vi "main.vi"() -> ()   [LabVIEW 2023]
uses:
  Enum.ctl
  typeDef/enum mesure.ctl
  Desktop/Open_device_2018.llb/Select_Instr.ctl
panel:
  in  "VISA resource name":refnum<visa-resource-name>
  out "?":T1
  out "Horizontal Progress Bar":u8(slide) scale=0.0..100.0
  in  "Exit program":bool
  in  "Start measure":bool
  in  "Pause measure":bool
  in  "Save As Button":bool
  in  "Sample distribution for graph":enum32{"Logarytmic", "Linear"}(radio)
  out "XY Graph":cluster{"X":dbl, "Y":dbl}[](graph)
  in  "Sample distribution":enum32{"Logarytmic", "Linear"}(radio)
  in  "Density distribution":dbl
  in  "Amplitude":dbl
  in  "Stop frequency":dbl
  in  "Start frequency":dbl
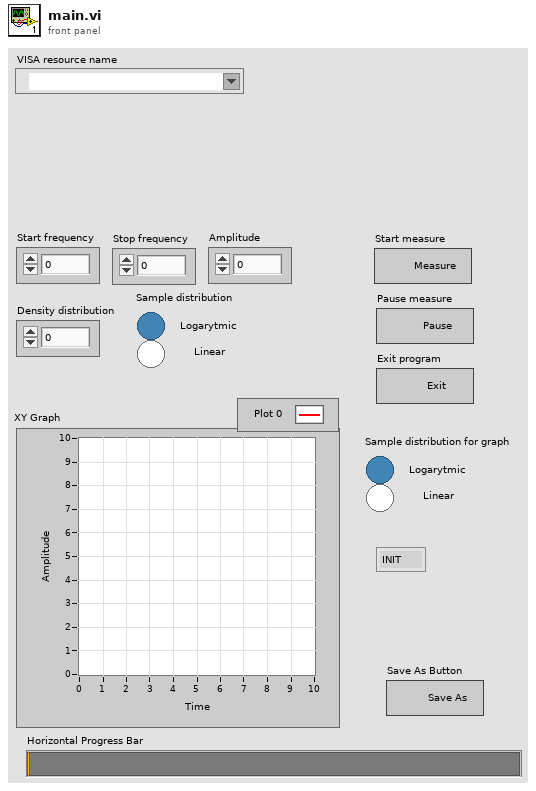
[diagram p1: front panel]
types:
  T1 = typedef "Enum.ctl" = enum16{"INIT", "IDLE", "SAVE", "CONN_TO_DEV", "MEASURE", "END", "CONN_TO_COM"}
  T2 = cluster{"COM_OK":bool, "MEASURE":bool, "komutator":refnum<visa-resource-name>, "generator":refnum<visa-resource-name>, "miernik":refnum<visa-resource-name>}
  T3 = typedef "enum mesure.ctl" = enum16{"Set_gen", "Obj_1", "Obj_2", "Obj_3", "Obj_4", "Obj_5"}
  T4 = typedef "Select_Instr.ctl" = string
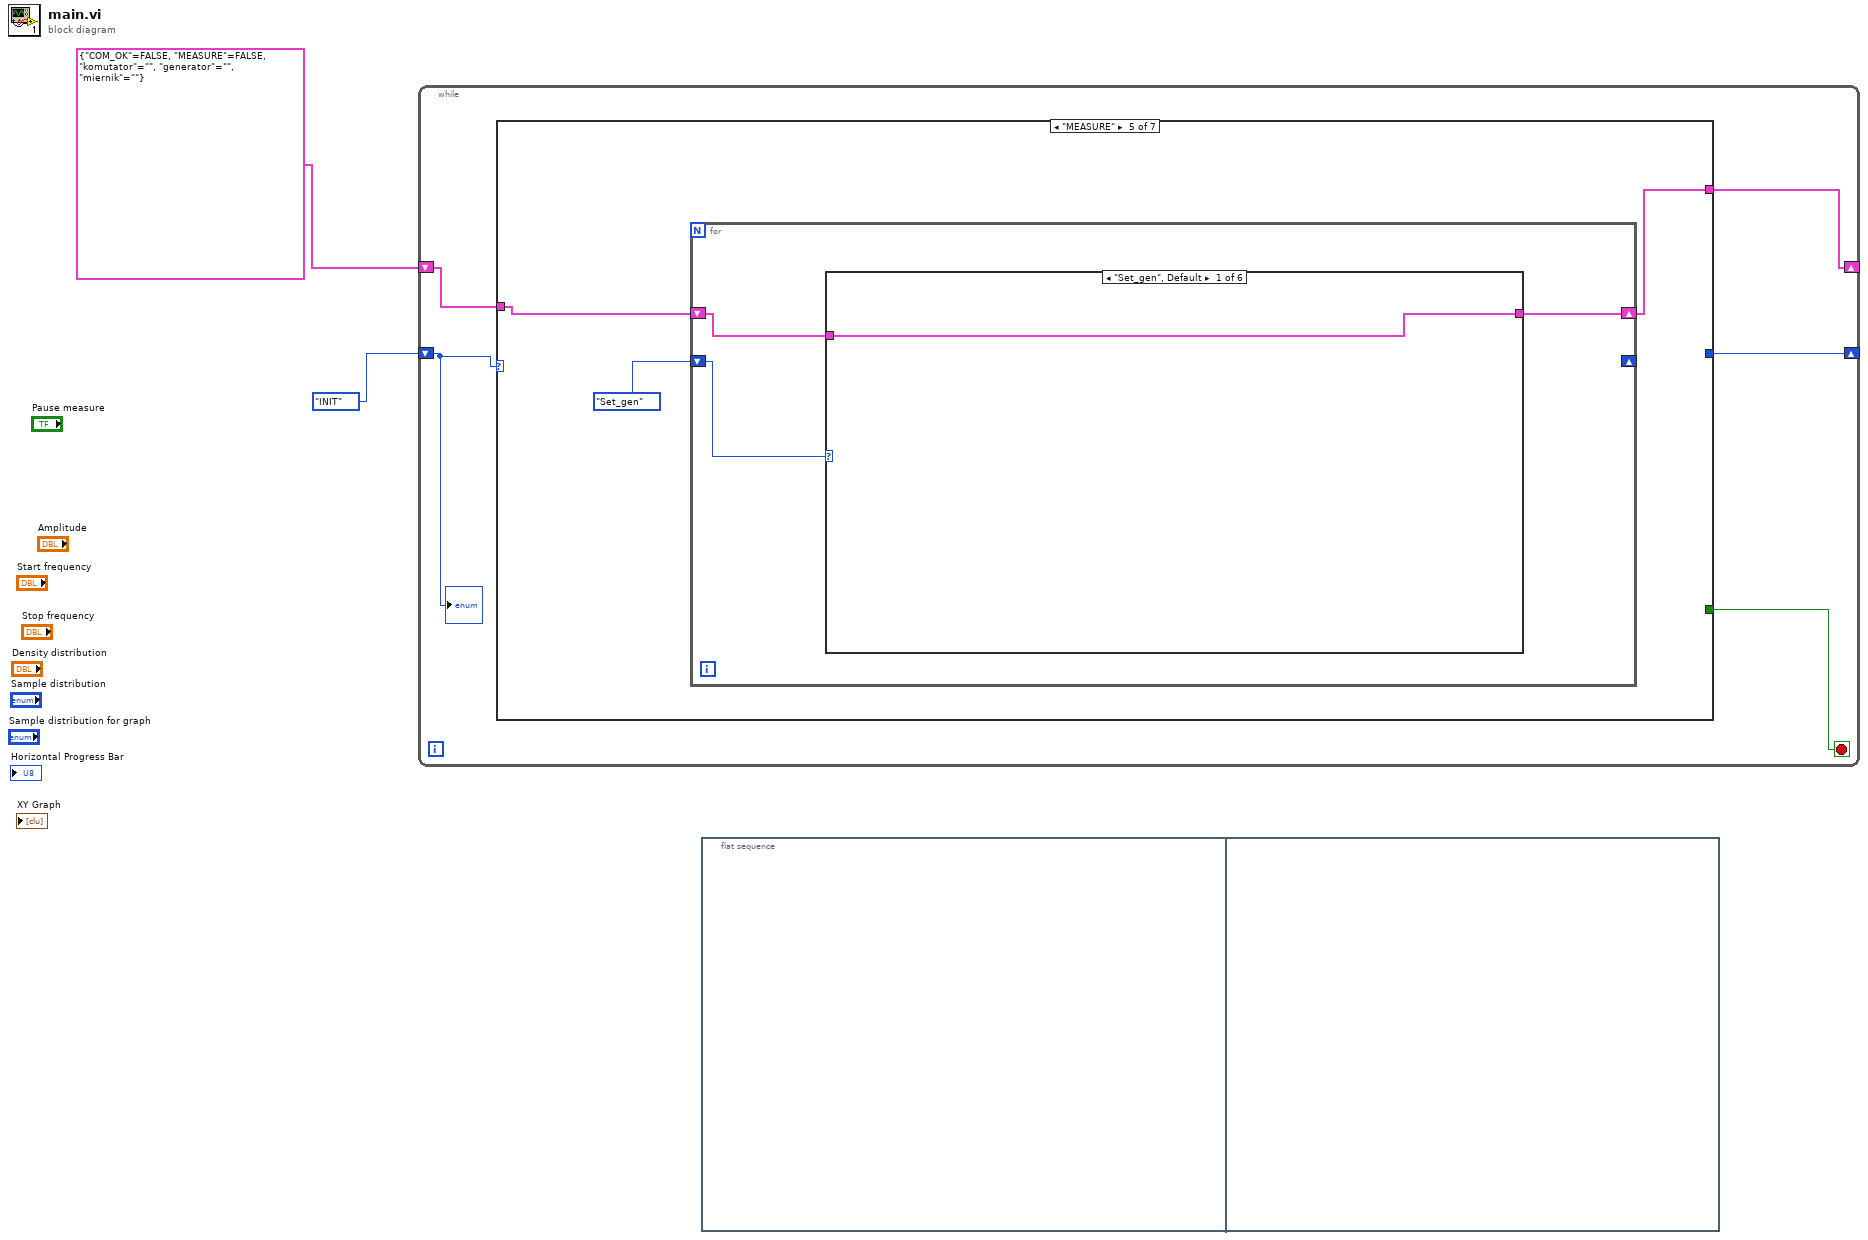
[diagram p0: block diagram]
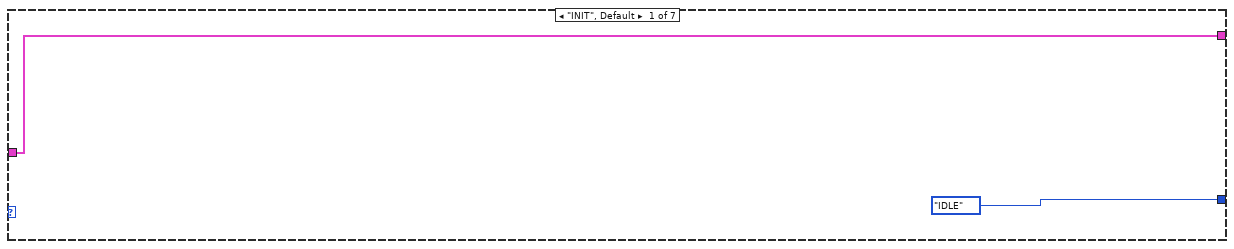
[diagram p2: hidden frame]
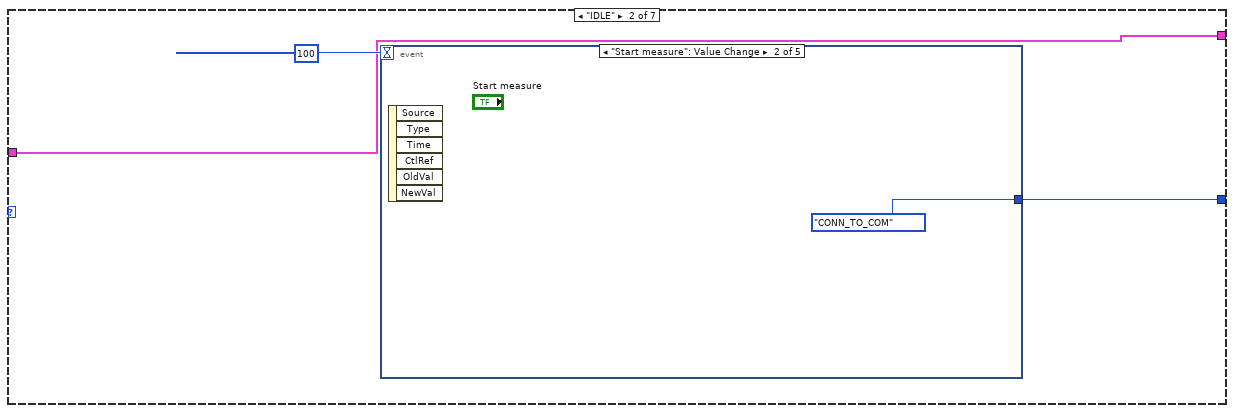
[diagram p3: hidden frame]
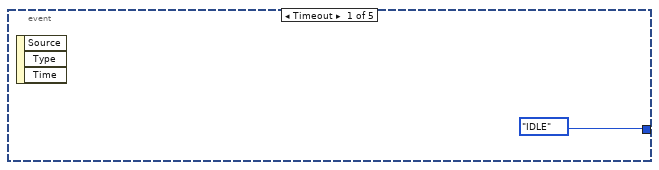
[diagram p4: hidden frame]
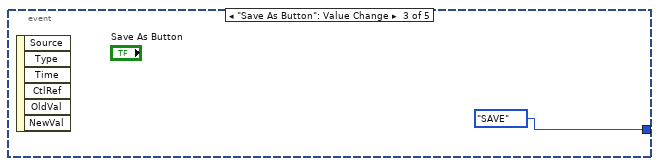
[diagram p5: hidden frame]
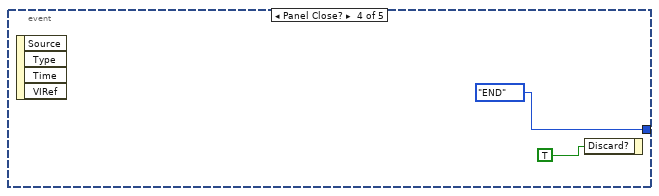
[diagram p6: hidden frame]
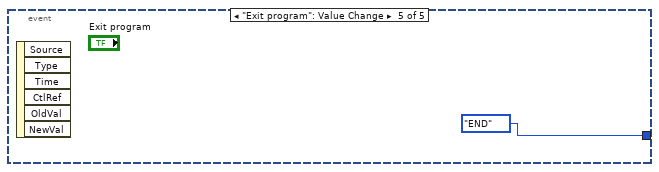
[diagram p7: hidden frame]
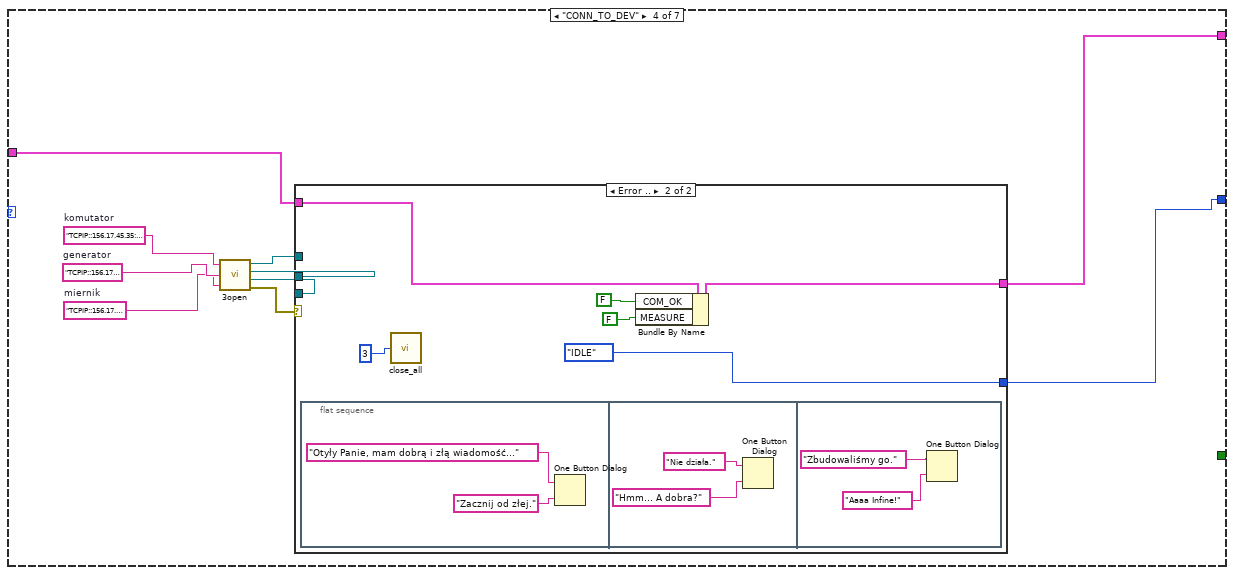
[diagram p9: hidden frame]
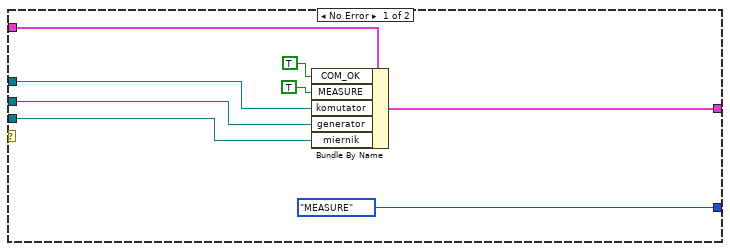
[diagram p10: hidden frame]
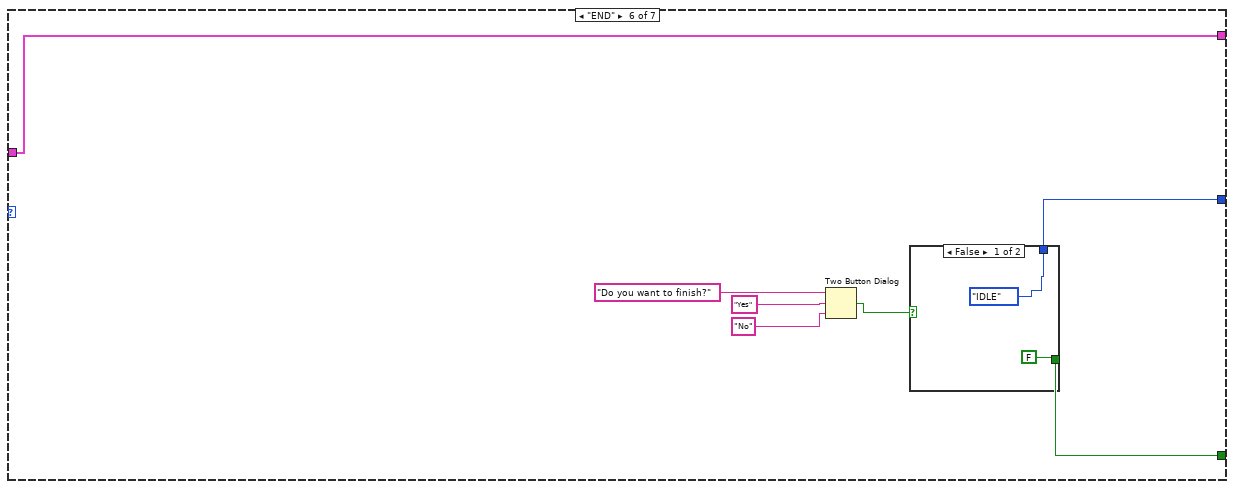
[diagram p16: hidden frame]
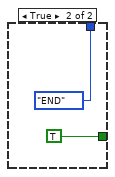
[diagram p17: hidden frame]
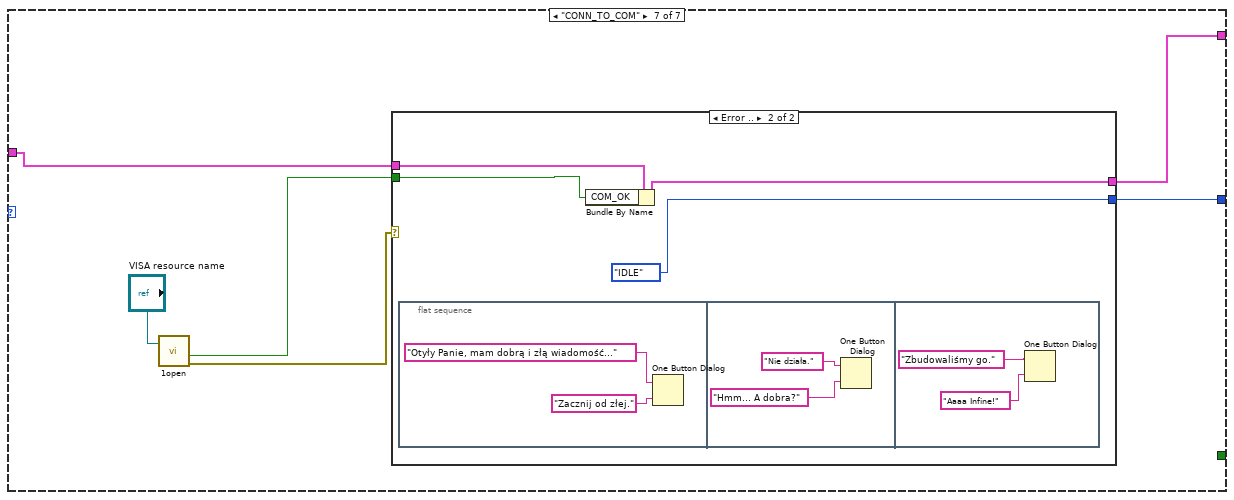
[diagram p18: hidden frame]
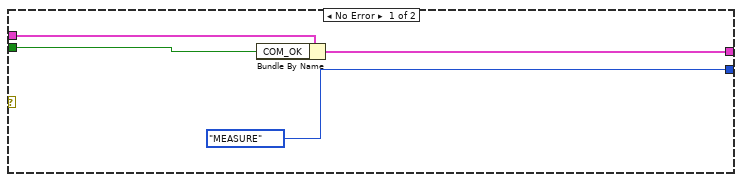
[diagram p19: hidden frame]
diagram:
  n1 = while {
    shift-right: [w5] -> _
    shift-left: Enum."INIT" -> [w7]
    shift-right: [w3] -> _
    shift-left: T2 {"COM_OK"=FALSE, "MEASURE"=FALSE, "komutator"="", "generator"="", "miernik"=""} -> [w4]
    stop <- w6 stop-if-true
    n2 = case shown="\"MEASURE\"" w7 {
      tunnel: [_ _ _ _ _ w59 _] -> w6
      tunnel: [Enum."IDLE" w12 _ w20 _ w58 w68] -> w5
      tunnel: w4 -> [w8 w10 w19 w25 w51 w57 w71]
      tunnel: [w8 w10 w19 w24 w50 w57 w69] -> w3
      frame "INIT", Default {
      }
      frame "IDLE" {
        n3 = event shown="[1] \"Start measure\": Value Change" {
          selector: _ -> [_ _ _ _ _]
          dyn-events: _ -> [_ _ _ _ _]
          timeout: 100 -> [_ _ _ _ _]
          tunnel: [Enum."IDLE" Enum."CONN_TO_COM" Enum."SAVE" Enum."END" Enum."END"] -> w12
          event Timeout {
            n4 = event-data() -> ()  [unwired: 1 in, 3 out]
          }
          event "Start measure": Value Change {
            n5 = event-data() -> ()  [unwired: 1 in, 6 out]
          }
          event "Save As Button": Value Change {
            n6 = event-data() -> ()  [unwired: 1 in, 6 out]
          }
          event Panel Close? {
            n7 = event-data() -> ()  [unwired: 1 in, 4 out]
            n8 = event-data("Discard?"=TRUE) -> ()  [unwired: 1 in, 1 out]
          }
          event "Exit program": Value Change {
            n9 = event-data() -> ()  [unwired: 1 in, 6 out]
          }
        }
      }
      frame "SAVE" {
      }
      frame "CONN_TO_DEV" {
        w27 = T4 "TCPIP::156.17.45.35::inst27::INSTR"  # miernik
        w28 = T4 "TCPIP::156.17.45.35::inst25::INSTR"  # generator
        w29 = T4 "TCPIP::156.17.45.35::inst104::INSTR"  # komutator
        n10 = call "3open.vi"("VISA resource name 1"=w29, "VISA resource name 2"=w28, "VISA resource name 3"=w27) -> ("VISA dup name 1"=w23:refnum<visa-resource-name>, "VISA dup name 2"=w22:refnum<visa-resource-name>, "VISA dup name 3"=w21:refnum<visa-resource-name>, "error out"=w26:errorcluster)  [unwired: 1 out]
        n11 = case shown="Error .." w26 {
          tunnel: w25 -> [w37 w43]
          tunnel: [w36 w42] -> w24
          tunnel: w23 -> [w35 _]
          tunnel: w22 -> [w34 _]
          tunnel: w21 -> [w33 _]
          tunnel: [Enum."MEASURE" Enum."IDLE"] -> w20
          frame No Error {
            n12 = Bundle By Name(cluster=w37, "COM_OK"=TRUE, "MEASURE"=TRUE, "komutator"=w35, "generator"=w34, "miernik"=w33) -> (w36:T2)
          }
          frame Error {
            n13 = flat-sequence {
              frame #0 {
                n14 = One Button Dialog(message="Otyły Panie, mam dobrą i złą wiadomość...", button name ("OK")="Zacznij od złej.") -> ()  [unwired: 1 out]
              }
              frame #1 {
                n15 = One Button Dialog(message="Nie działa.", button name ("OK")="Hmm... A dobra?") -> ()  [unwired: 1 out]
              }
              frame #2 {
                n16 = One Button Dialog(message="Zbudowaliśmy go.", button name ("OK")="Aaaa Infine!") -> ()  [unwired: 1 out]
              }
            }
            n17 = call "close_all.vi"("Dummy\n(for dataflow)"=3 ("Dummy\n(for dataflow)")) -> ()  [unwired: 1 out]
            n18 = Bundle By Name(cluster=w43, "COM_OK"=FALSE, "MEASURE"=FALSE) -> (w42:T2)
          }
        }
      }
      frame "MEASURE" {
        n19 = for {
          shift-right: _ -> [_]
          shift-left: enum_mesure."Set_gen" -> [w55]
          shift-right: [w54] -> w50
          shift-left: w51 -> [w53]
          n20 = case shown="\"Set_gen\", Default" w55 {
            tunnel: [w56 _ _ _ _ _] -> w54
            tunnel: w53 -> [w56 _ _ _ _ _]
            frame "Set_gen", Default {
            }
            frame "Obj_1" {
            }
            frame "Obj_2" {
            }
            frame "Obj_3" {
            }
            frame "Obj_4" {
            }
            frame "Obj_5" {
            }
          }
        }
      }
      frame "END" {
        n21 = Two Button Dialog(message="Do you want to finish?", 1:"No" ("F button name (\"Cancel\")"), 2:"Yes" ("T button name (\"OK\")")) -> (T button?=w63:bool)
        n22 = case shown="False" w63 {
          tunnel: [FALSE TRUE] -> w59
          tunnel: [Enum."IDLE" Enum."END"] -> w58
          frame False {
          }
          frame True {
          }
        }
      }
      frame "CONN_TO_COM" {
        n23 = call "1open.vi"("VISA resource name"="VISA resource name") -> ("Open OK (true)"=w70:bool, "error out"=w73:errorcluster)  [unwired: 1 in, 2 out]
        n24 = case shown="Error .." w73 {
          tunnel: w71 -> [w77 w81]
          tunnel: w70 -> [w76 w79]
          tunnel: [w75 w80] -> w69
          tunnel: [Enum."MEASURE" Enum."IDLE"] -> w68
          frame No Error {
            n25 = Bundle By Name(cluster=w77, "COM_OK"=w76) -> (w75:T2)
          }
          frame Error {
            n26 = flat-sequence {
              frame #0 {
                n27 = One Button Dialog(message="Otyły Panie, mam dobrą i złą wiadomość...", button name ("OK")="Zacznij od złej.") -> ()  [unwired: 1 out]
              }
              frame #1 {
                n28 = One Button Dialog(message="Nie działa.", button name ("OK")="Hmm... A dobra?") -> ()  [unwired: 1 out]
              }
              frame #2 {
                n29 = One Button Dialog(message="Zbudowaliśmy go.", button name ("OK")="Aaaa Infine!") -> ()  [unwired: 1 out]
              }
            }
            n30 = Bundle By Name(cluster=w81, "COM_OK"=w79) -> (w80:T2)
          }
        }
      }
    }
    "?" <- w7
  }
  n31 = flat-sequence {
    frame #0 {
    }
    frame #1 {
    }
  }
